vi "CB Elevator Gravity Feedforward.vi"(7 "Motor ID":T1, 9 "G (gear ratio)":dbl, 10 "pulley radius (m)":dbl, 11 "mass (kg)":dbl) -> (3 "feedforward":dbl)   [LabVIEW 2020]
uses:
  Motors/CB Motor ID.ctl
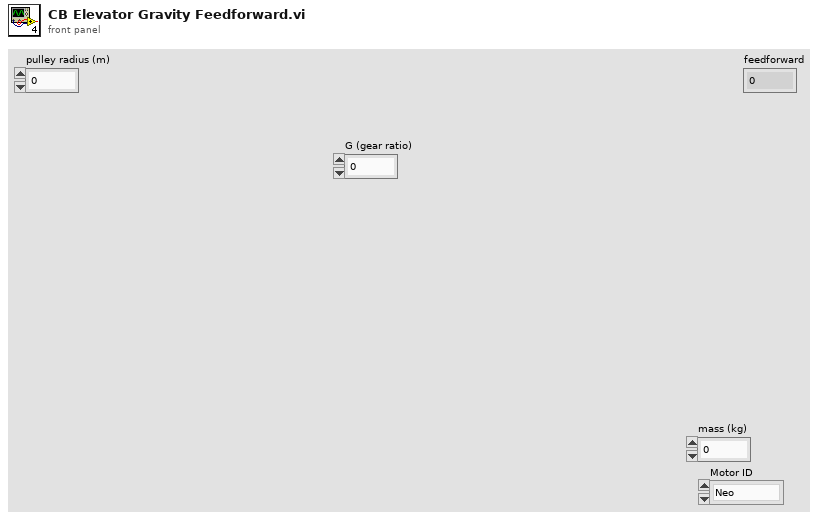
[diagram p1: front panel]
types:
  T1 = typedef "CB Motor ID.ctl" = enum16{"Neo", "Neo 550", "Falcon 500", "775pro"}
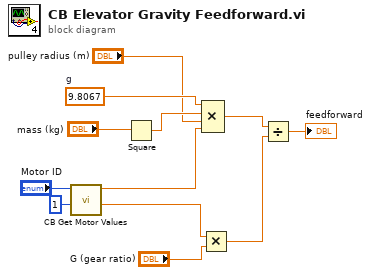
[diagram p0: block diagram]
diagram:
  w9 = 9.8067  # g
  n1 = call "CB Get Motor Values.vi"("num motors"=1, "Motor ID"="Motor ID") -> ("Kt"=w3:dbl, "R"=w6:dbl)  [unwired: 6 in, 2 out]
  n2 = Square(x="mass (kg)") -> (x^2=w8:dbl)
  n3 = Multiply(x=w3, y="G (gear ratio)") -> (x*y=w2:dbl)
  n4 = Compound Arithmetic op=MULTIPLY(w9, w8, "pulley radius (m)", w6) -> (w5:dbl)
  n5 = Divide(x=w5, y=w2) -> (x/y=→"feedforward":dbl)
